vi "Apply Stamp Precheck.vi"(8 "error in (no error)":errorcluster, 9 "Slot Number":i32, 10 "Chuck Number":i32, 11 "GrabberTool Class in":refnum<class "GrabberTool Class.lvclass">) -> (0 "error out":errorcluster, 3 "GrabberTool Class out":refnum<class "GrabberTool Class.lvclass">)   [LabVIEW 2011, in "GrabberTool Class.lvclass"]
uses:
  GrabberTool Class.lvclass
  WorkTable Class/WorkTable Class.lvclass
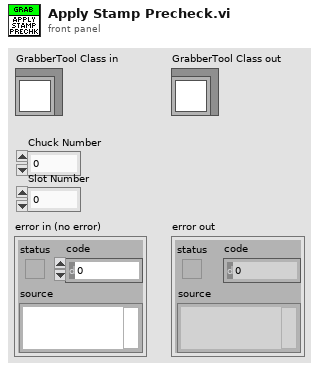
[diagram p1: front panel]
types:
  T1 = typedef "Worktable_Module Slot.ctl" = cluster{"Slot State":enum16{"Empty", "Unglued", "Stamped", "PartOnTop", "Weighted", "Unpotted", "Potted"}, "BBM Type":enum16{"None", "BBM", "GlassSlide"}, "HDI Type":enum16{"None", "HDI", "Polyimide"}, "Vacuum Channel":u8, "Location/Orientation BBM":T2, "Location/Orientation HDI":T2, "S/N":string}
  T2 = typedef "Position_Orientation.ctl" = cluster{"Center":refnum<class "Vec3d Class.lvclass">, "Orientation":refnum<class "Orient3d Class.lvclass">}
  T3 = enum16{"Empty", "Unglued", "Stamped", "PartOnTop", "Weighted", "Unpotted", "Potted"}
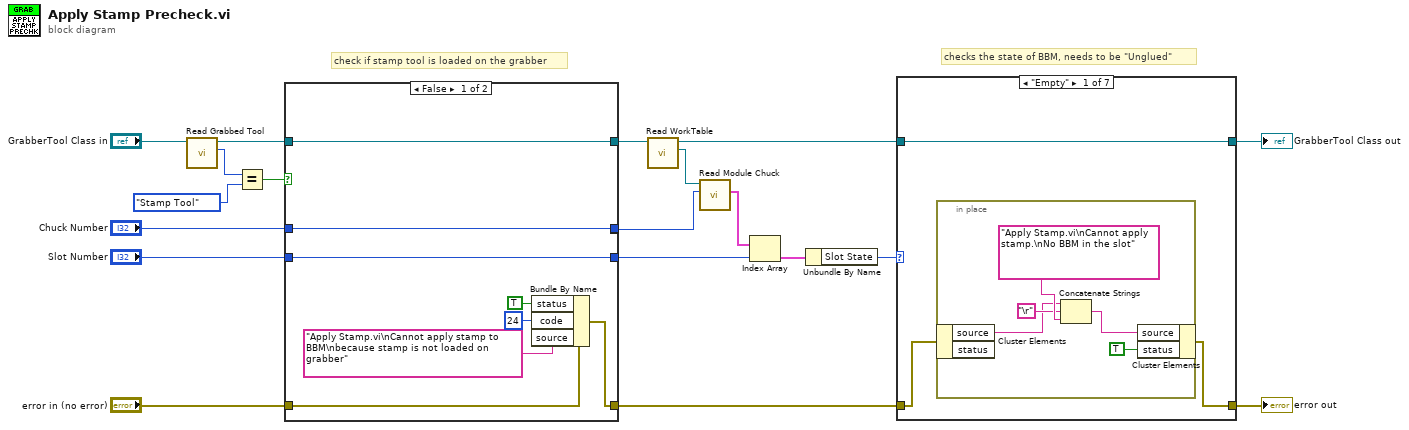
[diagram p0: block diagram]
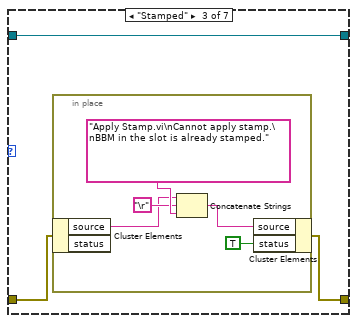
[diagram p3: hidden frame]
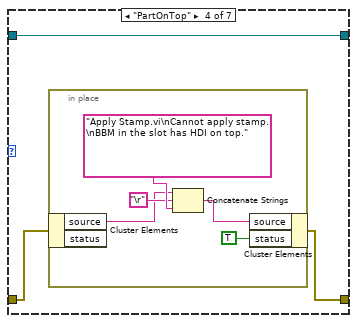
[diagram p4: hidden frame]
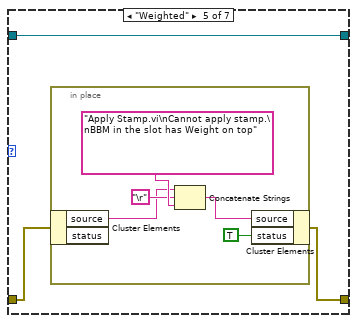
[diagram p5: hidden frame]
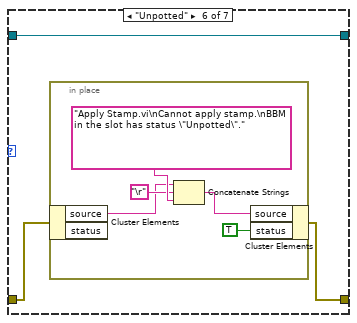
[diagram p6: hidden frame]
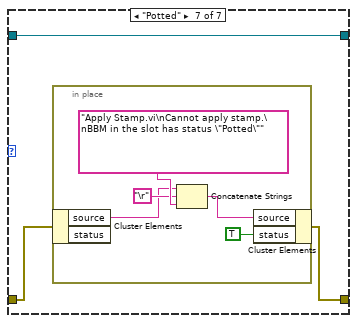
[diagram p7: hidden frame]
diagram:
  # "checks the state of BBM, needs to be \"Unglued\""
  # "check if stamp tool is loaded on the grabber"
  n1 = call "Read Grabbed Tool.vi"("GrabberTool Class in"="GrabberTool Class in") -> ("Grabbed Tool"=w18:enum16{"Weight Tool", "Stamp Tool", "Nothing"}, "GrabberTool Class out"=w15:refnum<class "GrabberTool Class.lvclass">)  [unwired: 8 in, 1 out]
  n2 = Equal?(x=w18, y=enum16{"Weight Tool", "Stamp Tool", "Nothing"}."Stamp Tool" ("Grabbed Tool")) -> (x = y?=w16:bool)
  n3 = case shown="False" w16 {
    tunnel: [w20 w30] -> w3
    tunnel: [w27 w31] -> w11
    tunnel: w15 -> [w27 w31]
    tunnel: "error in (no error)" -> [w21 w30]
    tunnel: "Chuck Number" -> [w26 w28]
    tunnel: [w26 w28] -> w9
    tunnel: [_ w28] -> _
    tunnel: "Slot Number" -> [w25 w29]
    tunnel: [w25 w29] -> w7
    frame False {
      n4 = Bundle By Name(cluster=w21, "status"=TRUE, "code"=24, "source"="Apply Stamp.vi\nCannot apply stamp to BBM\nbecause stamp is not loaded on grabber") -> (w20:errorcluster)
    }
    frame True {
    }
  }
  n5 = call-dynamic "Read WorkTable.vi"("Gantry Class in"=w11) -> ("WorkTable Class.lvclass"=w10:refnum<class "WorkTable Class.lvclass">, "Gantry Class out"=w4:refnum<class "GrabberTool Class.lvclass">)  [unwired: 8 in, 1 out]
  n6 = call-dynamic "Read Module Chuck.vi"("index"=w9, "WorkTable in"=w10) -> ("Module Slots"=w8:T1[])  [unwired: 7 in, 2 out]
  n7 = Index Array(array=w8, index=w7) -> (element=w6:T1)
  n8 = Unbundle By Name(w6) -> ("Slot State"=w5:T3)
  n9 = case shown="\"Empty\"" w5 {
    tunnel: w4 -> [w34 w41 w44 w52 w58 w66 w74]
    tunnel: [w34 w41 w44 w52 w58 w66 w74] -> w2
    tunnel: w3 -> [w33 w40 w42 w51 w60 w68 w76]
    tunnel: [w32 w40 w43 w50 w59 w67 w75] -> w1
    frame "Empty" {
      n10 = in-place {
        n11 = in-place-cluster #1(w33) -> ("source"=w36:string)  [unwired: 1 out]
        n12 = Concatenate Strings(w36, "\r", "Apply Stamp.vi\nCannot apply stamp.\nNo BBM in the slot" ("string")) -> (w37:string)
        n13 = in-place-cluster #1("source"=w37, "status"=TRUE) -> (w32:errorcluster)
      }
    }
    frame "Unglued" {
    }
    frame "Stamped" {
      n14 = in-place {
        n15 = in-place-cluster #2(w42) -> ("source"=w46:string)  [unwired: 1 out]
        n16 = Concatenate Strings(w46, "\r", "Apply Stamp.vi\nCannot apply stamp.\nBBM in the slot is already stamped." ("string")) -> (w47:string)
        n17 = in-place-cluster #2("source"=w47, "status"=TRUE) -> (w43:errorcluster)
      }
    }
    frame "PartOnTop" {
      n18 = in-place {
        n19 = in-place-cluster #3(w51) -> ("source"=w54:string)  [unwired: 1 out]
        n20 = Concatenate Strings(w54, "\r", "Apply Stamp.vi\nCannot apply stamp.\nBBM in the slot has HDI on top." ("string")) -> (w55:string)
        n21 = in-place-cluster #3("source"=w55, "status"=TRUE) -> (w50:errorcluster)
      }
    }
    frame "Weighted" {
      n22 = in-place {
        n23 = in-place-cluster #4(w60) -> ("source"=w62:string)  [unwired: 1 out]
        n24 = Concatenate Strings(w62, "\r", "Apply Stamp.vi\nCannot apply stamp.\nBBM in the slot has Weight on top" ("string")) -> (w63:string)
        n25 = in-place-cluster #4("source"=w63, "status"=TRUE) -> (w59:errorcluster)
      }
    }
    frame "Unpotted" {
      n26 = in-place {
        n27 = in-place-cluster #5(w68) -> ("source"=w70:string)  [unwired: 1 out]
        n28 = Concatenate Strings(w70, "\r", "Apply Stamp.vi\nCannot apply stamp.\nBBM in the slot has status \"Unpotted\"." ("string")) -> (w71:string)
        n29 = in-place-cluster #5("source"=w71, "status"=TRUE) -> (w67:errorcluster)
      }
    }
    frame "Potted" {
      n30 = in-place {
        n31 = in-place-cluster #6(w76) -> ("source"=w78:string)  [unwired: 1 out]
        n32 = Concatenate Strings(w78, "\r", "Apply Stamp.vi\nCannot apply stamp.\nBBM in the slot has status \"Potted\"" ("string")) -> (w79:string)
        n33 = in-place-cluster #6("source"=w79, "status"=TRUE) -> (w75:errorcluster)
      }
    }
  }
  "error out" <- w1
  "GrabberTool Class out" <- w2
